vi "Get Freq Correction.vi"(8 "error in (no error)":errorcluster, 11 "RTL-SDR in":refnum<class "RTL-SDR.lvclass">) -> (0 "error out":errorcluster, 2 "Frequency Correction (ppm)":i32, 3 "RTL-SDR out":refnum<class "RTL-SDR.lvclass">)   [LabVIEW 2015, in "RTL-SDR.lvclass"]
uses:
  RTL-SDR.lvclass
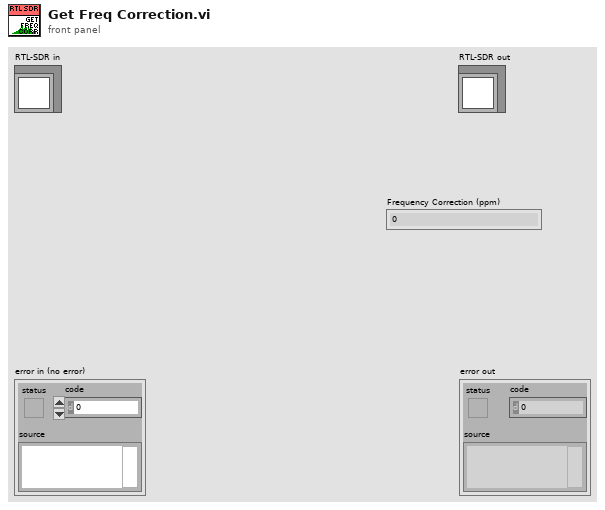
[diagram p1: front panel]
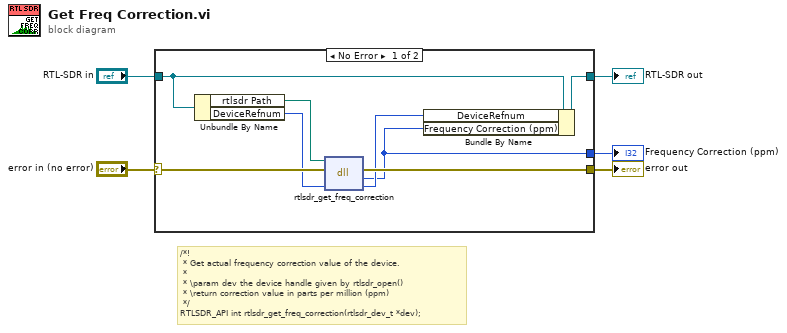
[diagram p0: block diagram]
diagram:
  # "/*!\n * Get actual frequency correction value of the device.\n *\n * \\param dev the device handle given by rtlsdr_open()\n * \\return correction value in parts per million (ppm)\n */\nRTLSDR_API int rtlsdr_get_freq_correction(rtlsdr_dev_t *dev);"
  n1 = case shown="No Error" "error in (no error)" {
    selector: "error in (no error)" -> [w13 w15]
    tunnel: [w12 w15] -> w4
    tunnel: [w8 w14] -> w2
    tunnel: "RTL-SDR in" -> [w11 w14]
    tunnel: [w6 _] -> w1
    frame No Error {
      n2 = Unbundle By Name(w11) -> ("rtlsdr Path"=w10:path, "DeviceRefnum"=w9:u64)
      n3 = dll-call lib="C:/Users/Ivan/Desktop/D-23-09-24 (RTL-SDR)/Project (Pelleng-SDR)/RTL-SDR Class/dll/rtlsdr.*" fn="rtlsdr_get_freq_correction"(path in=w10, error in=w13, "DeviceRefnum"=w9) -> (error out=w12:errorcluster, "return type"=w6:i32, "DeviceRefnum"=w7:u64)  [unwired: 1 in, 1 out]
      n4 = Bundle By Name(cluster=w11, "DeviceRefnum"=w7, "Frequency Correction (ppm)"=w6) -> (w8:refnum<class "RTL-SDR.lvclass">)
    }
    frame Error {
    }
  }
  "error out" <- w4
  "RTL-SDR out" <- w2
  "Frequency Correction (ppm)" <- w1
